vi "AD7747_Convert_Hex_to_Cap.vi"(0 "Cap_Data":u8[][](array[numeric])=[[0, 0, 0, 0, 0, 0, 0, 0, 0, 0, 0, 0, 0, 0, 0, 0], [0, 0, 0, 0, 0, 0, 0, 0, 0, 0, 0, 0, 0, 0, 0, 0]] format="%.0x", 11 "error in (no error)":errorcluster) -> (3 "number":u32 format="%.0x", 4 "Cap":dbl, 6 "Reg1":u8 format="%.0x", 8 "Reg2":u8 format="%.0x", 10 "Reg3":u8 format="%.0x", 15 "error out":errorcluster)   [LabVIEW 2012]
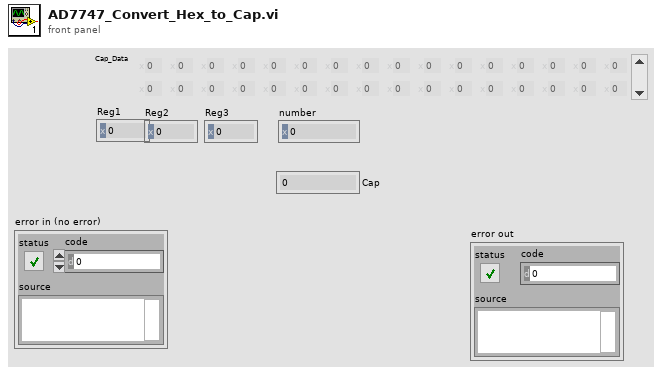
[diagram p1: front panel]
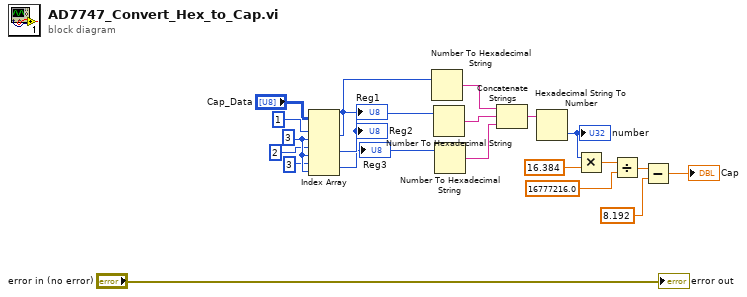
[diagram p0: block diagram]
diagram:
  w19 = 3 ("index (row)")
  n1 = Index Array(array="Cap_Data", index (row) #1=1 ("index (row)"), index (col) #1=w19, index (row) #2=2 ("index (row)"), index (col) #2=w19, index (row) #3=3 ("index (row)"), index (col) #3=w19) -> (element #1=w15:u8, element #2=w14:u8, element #3=w13:u8)
  "Reg1" <- w15
  "Reg2" <- w14
  "Reg3" <- w13
  n2 = Number To Hexadecimal String(2:w15) -> (0:w12:string)  [unwired: 1 in]
  n3 = Number To Hexadecimal String(2:w14) -> (0:w11:string)  [unwired: 1 in]
  n4 = Number To Hexadecimal String(2:w13) -> (0:w10:string)  [unwired: 1 in]
  n5 = Concatenate Strings(w12, w11, w10) -> (w9:string)
  n6 = Hexadecimal String To Number(string=w9) -> (number=w8:u32)  [unwired: 2 in, 1 out]
  "number" <- w8
  n7 = Multiply(x=w8, y=16.384) -> (x*y=w6:dbl)
  n8 = Divide(x=w6, y=16777216.0) -> (x/y=w3:dbl)
  n9 = Subtract(x=w3, y=8.192) -> (x-y=→"Cap":dbl)
  "error out" <- "error in (no error)"
